vi "Delete Subsystems.vi"(8 "error in (no error)":errorcluster, 10 "Subsystems":T1[](array[typedef]), 11 "System Name":string) -> (0 "error out":errorcluster)   [LabVIEW 2024]
doc: "Deletes subsystems in the shared variable engine."
uses:
  Controls/Server/Subsystem Configuration.ctl
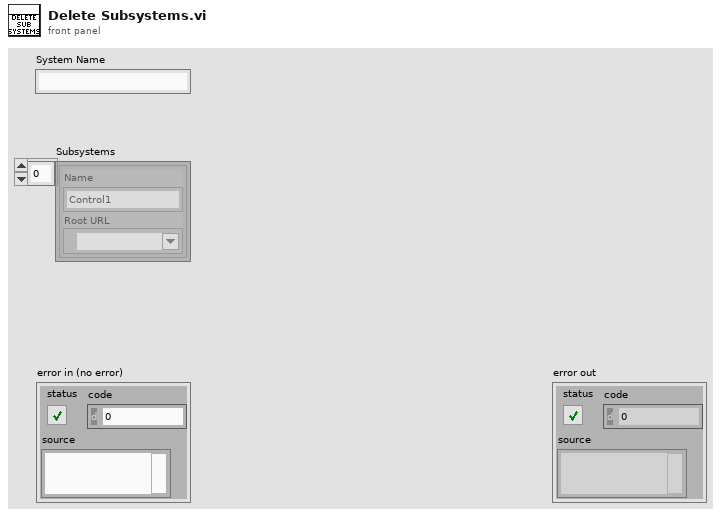
[diagram p1: front panel]
types:
  T1 = typedef "Subsystem Configuration.ctl" = cluster{"Name":string, "Root URL":refnum<k21>}
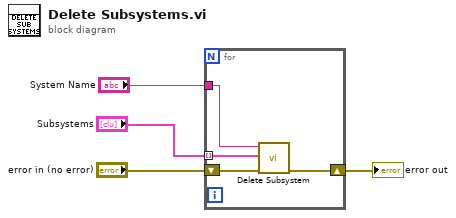
[diagram p0: block diagram]
diagram:
  n1 = for {
    tunnel: "Subsystems" -> [w5] mode=indexing
    shift-right: [w7] -> w2
    shift-left: "error in (no error)" -> [w8]
    tunnel: "System Name" -> [w6]
    n2 = call "Delete Subsystem.vi"("error in (no error)"=w8, "Subsystem"=w5, "System Name"=w6) -> ("error out"=w7:errorcluster)  [unwired: 8 in]
  }
  "error out" <- w2
